vi "Refresh IP Channels.vi"(8 "error in (no error)":errorcluster, 9 "Main":string, 10 "GUID":string, 11 "Section Ref in":T1 format="%.0x") -> (0 "error out":errorcluster, 3 "Section Ref out":T1 format="%.0x")   [LabVIEW 2015, in "Engine Simulation Toolkit System Explorer.lvlib"]
uses:
  Engine Simulation Toolkit System Explorer.lvlib
  <vilib>/NI Veristand/Custom Device API/Custom Device Item Ref.ctl
  <vilib>/NI Veristand/Custom Device API/Get Item Property (String Array).vi
  <vilib>/NI Veristand/Custom Device Tools/Custom Device Utility Library/NI VeriStand - Search for All Items by GUID.vi
  Shared/Properties.vi
  <vilib>/NI Veristand/Custom Device API/Get Item Property (String).vi
  <vilib>/NI Veristand/Custom Device Tools/Custom Device Utility Library/Custom Device Utility Library.lvlib
  <vilib>/NI Veristand/Custom Device API/Custom Device API.lvlib
  Shared/Engine Simulation Toolkit Shared.lvlib
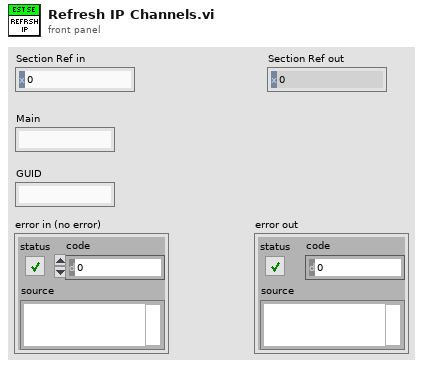
[diagram p1: front panel]
types:
  T1 = typedef "Custom Device API.lvlib/Custom Device Item Ref.ctl" = u64
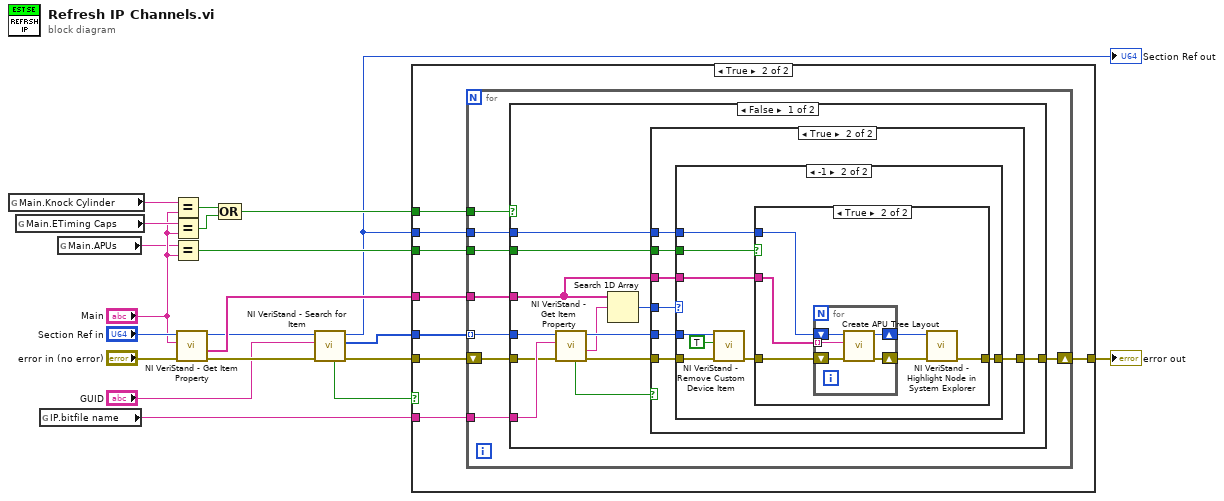
[diagram p0: block diagram]
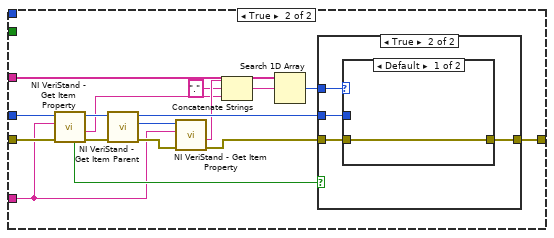
[diagram p6: hidden frame]
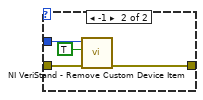
[diagram p8: hidden frame]
diagram:
  n1 = global read "Properties.vi" "Main.Knock Cylinder"() -> (w7:string)
  n2 = global read "Properties.vi" "Main.ETiming Caps"() -> (w8:string)
  n3 = global read "Properties.vi" "IP.bitfile name"() -> (w20:string)
  n4 = global read "Properties.vi" "Main.APUs"() -> (w3:string)
  n5 = Equal?(x=w7, y="Main") -> (x = y?=w6:bool)
  n6 = Equal?(x=w8, y="Main") -> (x = y?=w5:bool)
  n7 = Equal?(x=w3, y="Main") -> (x = y?=w2:bool)
  n8 = call-poly <vilib>:"NI VeriStand - Get Item Property.vi"("error in (no error)"="error in (no error)", "Property Name"="Main", "Item Ref in"="Section Ref in") -> ("error out"=w10:errorcluster, "Value"=w15:string[], "Item Ref out"=w11:T1)  [unwired: 5 in, 1 out]
  n9 = Compound Arithmetic op=OR(w6, w5) -> (w14:bool)
  n10 = call-poly <vilib>:"NI VeriStand - Search for Item.vi"("error in"=w10, "Item GUID"="GUID", "Section Ref in"=w11) -> ("error out"=w16:errorcluster, "Item Refs"=w17:T1[], "Section Ref out"=w1:T1, "Found"=w19:bool)  [unwired: 5 in]
  "Section Ref out" <- w1
  n11 = case shown="True" w19 {
    tunnel: w16 -> [w21 w29]
    tunnel: w17 -> [_ w28]
    tunnel: w20 -> [_ w27]
    tunnel: [w21 w26] -> w18
    tunnel: w15 -> [_ w25]
    tunnel: w14 -> [_ w24]
    tunnel: w2 -> [_ w23]
    tunnel: w1 -> [_ w22]
    frame False {
    }
    frame True {
      n12 = for {
        tunnel: w27 -> [w37]
        tunnel: w28 -> [w35] mode=indexing
        shift-right: [w33] -> w26
        shift-left: w29 -> [w36]
        tunnel: w25 -> [w34]
        tunnel: w24 -> [w32]
        tunnel: w23 -> [w31]
        tunnel: w22 -> [w30]
        n13 = case shown="False" w32 {
          tunnel: w37 -> [w49 w83]
          tunnel: w36 -> [w48 w95]
          tunnel: w35 -> [w47 w94]
          tunnel: w34 -> [w38 w93]
          tunnel: [w42 w89] -> w33
          tunnel: w31 -> [w40 _]
          tunnel: w30 -> [w39 _]
          frame False {
            n14 = call-poly <vilib>:"NI VeriStand - Get Item Property.vi"("error in (no error)"=w48, "Property Name"=w49, "Item Ref in"=w47) -> ("error out"=w46:errorcluster, "Value"=w41:string, "Item Ref out"=w43:T1, "Found?"=w45:bool)  [unwired: 5 in]
            n15 = Search 1D Array(1D array=w38, element=w41) -> (index of element=w44:i32)  [unwired: 1 in]
            n16 = case shown="True" w45 {
              tunnel: w46 -> [w50 w56]
              tunnel: w44 -> [_ w57]
              tunnel: w43 -> [_ w55]
              tunnel: [w50 w54] -> w42
              tunnel: w40 -> [_ w51]
              tunnel: w39 -> [_ w53]
              tunnel: w38 -> [_ w52]
              frame False {
              }
              frame True {
                n17 = case shown="-1" w57 {
                  tunnel: w56 -> [w58 w66]
                  tunnel: w55 -> [_ w65]
                  tunnel: [w58 w62] -> w54
                  tunnel: w53 -> [_ w61]
                  tunnel: w52 -> [_ w60]
                  tunnel: w51 -> [_ w59]
                  frame Default {
                  }
                  frame -1 {
                    n18 = call <vilib>:"NI VeriStand - Remove Custom Device Item.vi"("error in (no error)"=w66, "Force Delete (F)"=TRUE, "Item Ref in"=w65) -> ("error out"=w63:errorcluster)  [unwired: 7 in, 1 out]
                    n19 = case shown="True" w59 {
                      tunnel: w63 -> [w67 w73]
                      tunnel: [w67 w68] -> w62
                      tunnel: w61 -> [_ w72]
                      tunnel: w60 -> [_ w71]
                      frame False {
                      }
                      frame True {
                        n20 = for {
                          shift-right: [w77] -> w69
                          shift-left: w73 -> [w78]
                          tunnel: w71 -> [w75] mode=indexing
                          shift-right: [w74] -> w70
                          shift-left: w72 -> [w76]
                          n21 = call "Create APU Tree Layout.vi"("error in (no error)"=w78, "engine name"=w75, "Section Ptr"=w76) -> ("error out"=w77:errorcluster, "Section Ptr dup"=w74:T1)  [unwired: 6 in, 1 out]
                        }
                        n22 = call <vilib>:"NI VeriStand - Highlight Node in System Explorer.vi"("error in (no error)"=w69, "Item Ref in"=w70) -> ("error out"=w68:errorcluster)  [unwired: 8 in, 1 out]
                      }
                    }
                  }
                }
              }
            }
          }
          frame True {
            n23 = call-poly <vilib>:"NI VeriStand - Get Item Property.vi"("error in (no error)"=w95, "Property Name"=w83, "Item Ref in"=w94) -> ("error out"=w85:errorcluster, "Value"=w80:string, "Item Ref out"=w90:T1, "Found?"=w92:bool)  [unwired: 5 in]
            n24 = call <vilib>:"NI VeriStand - Get Item Parent.vi"("error in (no error)"=w85, "Item Ref in"=w90) -> ("error out"=w84:errorcluster, "Parent Ref"=w86:T1, "Item Ref out"=w88:T1)  [unwired: 6 in, 1 out]
            n25 = call-poly <vilib>:"NI VeriStand - Get Item Property.vi"("error in (no error)"=w84, "Property Name"=w83, "Item Ref in"=w86) -> ("error out"=w87:errorcluster, "Value"=w82:string)  [unwired: 5 in, 2 out]
            n26 = Concatenate Strings(w82, "." ("string"), w80) -> (w79:string)
            n27 = Search 1D Array(1D array=w93, element=w79) -> (index of element=w91:i32)  [unwired: 1 in]
            n28 = case shown="True" w92 {
              tunnel: w87 -> [w96 w99]
              tunnel: w91 -> [_ w100]
              tunnel: w88 -> [_ w98]
              tunnel: [w96 w97] -> w89
              frame False {
              }
              frame True {
                n29 = case shown="Default" w100 {
                  tunnel: w99 -> [w101 w105]
                  tunnel: w98 -> [_ w103]
                  tunnel: [w101 w104] -> w97
                  frame Default {
                  }
                  frame -1 {
                    n30 = call <vilib>:"NI VeriStand - Remove Custom Device Item.vi"("error in (no error)"=w105, "Force Delete (F)"=TRUE, "Item Ref in"=w103) -> ("error out"=w104:errorcluster)  [unwired: 7 in, 1 out]
                  }
                }
              }
            }
          }
        }
      }
    }
  }
  "error out" <- w18
